vi "DAQ- Steper 2.vi"(0 "Travel (Degree)":dbl=100.0, 1 "Loda based":bool, 5 "Mode":i32(ring)=10178 items=["Finite Samples"=10178, "Continuous Samples"=10123, "Hardware Timed Single Point"=12522], 7 "Home Done":bool, 9 "Speed d/s":dbl=10.0, 11 "error in":errorcluster) -> (6 "Task Done Bit":bool, 15 "error out":errorcluster)   [LabVIEW 2020]
uses:
  Project Setup/Globle Variable/GR_Servo.vi
  <vilib>/DAQmx/create/channels.llb/DAQmx Create Channel (CO-Pulse Generation-Frequency).vi
  <vilib>/DAQmx/configure/timing.llb/DAQmx Timing (Implicit).vi
  Galobal variable_TI.vi
panel:
  out "32bit integer":i32
  in  "Motor PPR":dbl=3600.0
  in  "Motor Gear Ratio":dbl=1.0
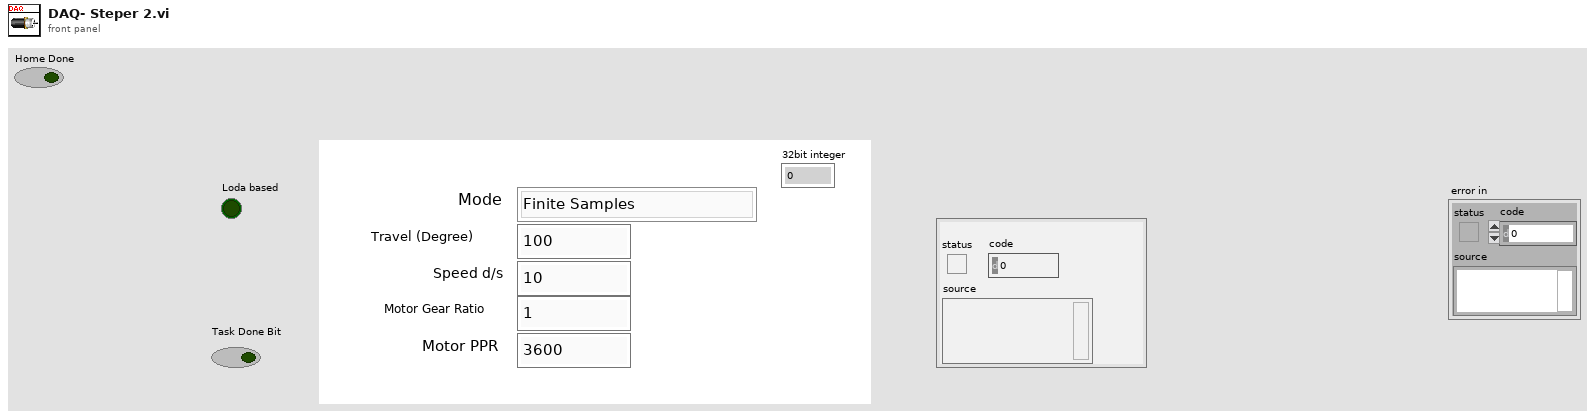
[diagram p1: front panel]
types:
  T1 = cluster{"MaxLoad ":dbl, "Min Load":dbl, "MaxDistance(mm)":dbl, "Min Distance(mm)":dbl, "Load Offset":dbl, "Model":string, "Difusser Code":string, "TFT Code ":string, "LVDT Offset":dbl}
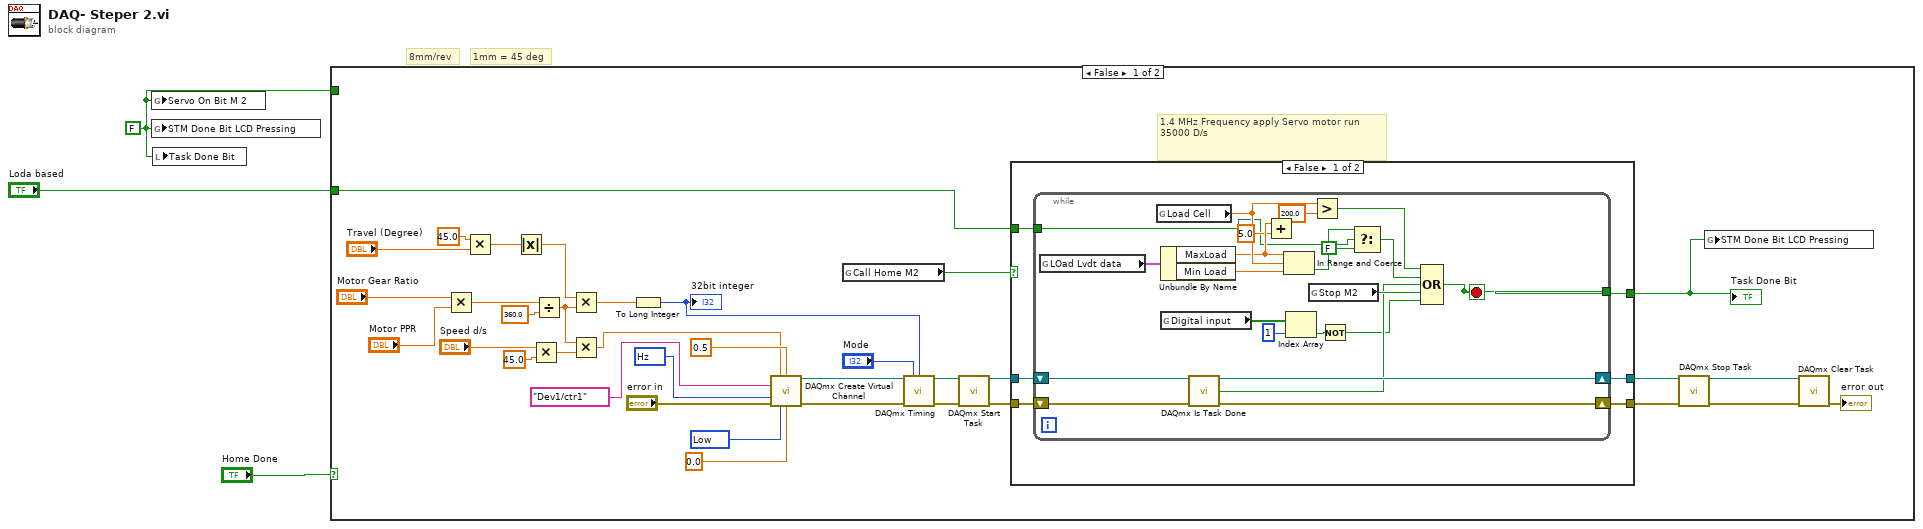
[diagram p0: block diagram]
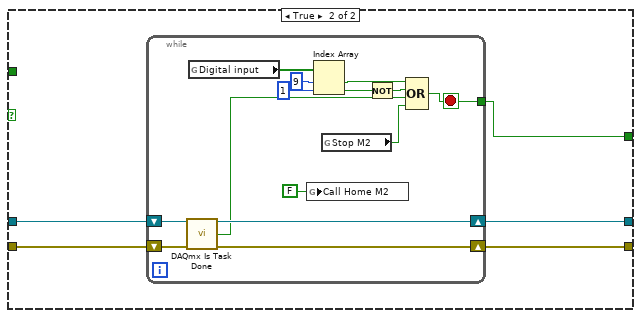
[diagram p2: hidden frame]
diagram:
  w3 = FALSE ("Servo On Bit M 2")
  # "1mm = 45 deg"
  # "8mm/rev"
  n1 = global write "GR_Servo.vi" "Servo On Bit M 2"(w3) -> ()
  n2 = global write "GR_Servo.vi" "STM Done Bit LCD Pressing"(w3) -> ()
  n3 = local write "Task Done Bit"(w3) -> ()
  n4 = case shown="False" "Home Done" {
    tunnel: w3 -> [_ _]
    tunnel: "Loda based" -> [w4 _]
    frame False {
      w18 = 10373 items=["Hz"=10373] ("units")
      w19 = 10214 items=["High"=10192, "Low"=10214] ("idle state")
      # "1.4 MHz Frequency apply Servo motor run \n35000 D/s"
      n5 = Multiply(x="Motor Gear Ratio", y="Motor PPR") -> (x*y=w28:dbl)
      n6 = Multiply(x=45.0, y="Travel (Degree)") -> (x*y=w16:dbl)
      n7 = Absolute Value(x=w16) -> (abs(x)=w27:dbl)
      n8 = Multiply(x="Speed d/s", y=45.0) -> (x*y=w13:dbl)
      n9 = Divide(x=w28, y=360.0) -> (x/y=w32:dbl)
      n10 = Multiply(x=w27, y=w32) -> (x*y=w17:dbl)
      n11 = Multiply(x=w32, y=w13) -> (x*y=w36:dbl)
      n12 = To Long Integer(number=w17) -> (32bit integer=w39:i32)
      "32bit integer" <- w39
      n13 = call-poly <vilib>:"DAQmx Create Virtual Channel.vi"("frequency"=w36, "duty cycle"=0.5, "counter"=tag "Dev1/ctr1", "units"=w18, "error in"="error in", "idle state"=w19, "initial delay"=0.0) -> ("task out"=w21:refnum<k21>, "error out"=w22:errorcluster)  [unwired: 7 in]
      n14 = global read "Galobal variable_TI.vi" "Call Home M2"() -> (w8:bool)
      n15 = call-poly <vilib>:"DAQmx Timing.vi"("task/channels in"=w21, "sample mode"="Mode", "samples per channel"=w39, "error in"=w22) -> ("task out"=w23:refnum<k21>, "error out"=w24:errorcluster)  [unwired: 10 in]
      n16 = call <vilib>:"DAQmx Start Task.vi"("task/channels in"=w23, "error in"=w24) -> ("task out"=w10:refnum<k21>, "error out"=w9:errorcluster)  [unwired: 12 in]
      n17 = case shown="False" w8 {
        tunnel: [w45 w69] -> w6
        tunnel: w10 -> [w44 w72]
        tunnel: [w43 w70] -> w7
        tunnel: w9 -> [w42 w71]
        tunnel: [w41 w68] -> w5
        tunnel: w4 -> [w40 _]
        frame False {
          n18 = while {
            shift-right: [w65] -> w43
            shift-left: w44 -> [w67]
            shift-right: [w66] -> w45
            shift-left: w42 -> [w64]
            tunnel: [w61] -> w41
            tunnel: w40 -> [w49]
            stop <- w61 stop-if-true
            n19 = global read "Galobal variable_TI.vi" "LOad Lvdt data"() -> (w56:T1)
            n20 = global read "Galobal variable_TI.vi" "Load Cell"() -> (w53:dbl)
            n21 = Unbundle By Name(w56) -> ("MaxLoad"=w52:dbl, "Min Load"=w55:dbl)
            n22 = global read "Galobal variable_TI.vi" "Digital input"() -> (w60:bool[])
            n23 = call <vilib>:"DAQmx Is Task Done.vi"("task/channels in"=w67, "error in"=w64) -> ("task out"=w65:refnum<k21>, "task done?"=w62:bool, "error out"=w66:errorcluster)  [unwired: 11 in]
            n24 = Add(x=w52, y=5.0) -> ()  [unwired: 1 out]
            n25 = In Range and Coerce(upper limit=w52, x=w53, lower limit=w55) -> (In Range?=w48:bool)  [unwired: 1 out]
            n26 = Index Array(array=w60, index=1) -> (element=w58:bool)
            n27 = global read "Galobal variable_TI.vi" "Stop M2"() -> (w63:bool)
            n28 = Greater?(x=w53, y=200.0) -> (0:w54:bool)
            n29 = Not(x=w58) -> (.not. x?=w57:bool)
            n30 = Select(t=w48, s=w49, f=FALSE) -> (s? t:f=w47:bool)
            n31 = Compound Arithmetic op=OR(w54, w47, w62, w63, w57) -> (w61:bool)
          }
        }
        frame True {
          n32 = while {
            shift-right: [w84] -> w70
            shift-left: w72 -> [w86]
            shift-right: [w85] -> w69
            shift-left: w71 -> [w83]
            tunnel: [w78] -> w68
            stop <- w78 stop-if-true
            n33 = call <vilib>:"DAQmx Is Task Done.vi"("task/channels in"=w86, "error in"=w83) -> ("task out"=w84:refnum<k21>, "task done?"=w79:bool, "error out"=w85:errorcluster)  [unwired: 11 in]
            n34 = global read "Galobal variable_TI.vi" "Digital input"() -> (w80:bool[])
            n35 = global write "Galobal variable_TI.vi" "Call Home M2"(FALSE ("Call Home M2")) -> ()
            n36 = Index Array(array=w80, index #1=9 ("index"), index #2=1 ("index")) -> (element #1=w75:bool, element #2=w74:bool)
            n37 = global read "Galobal variable_TI.vi" "Stop M2"() -> (w82:bool)
            n38 = Not(x=w74) -> (.not. x?=w73:bool)
            n39 = Compound Arithmetic op=OR(w75, w73, w79, w82) -> (w78:bool)
          }
        }
      }
      "Task Done Bit" <- w5
      n40 = call <vilib>:"DAQmx Stop Task.vi"("task/channels in"=w7, "error in"=w6) -> ("task out"=w25:refnum<k21>, "error out"=w35:errorcluster)  [unwired: 12 in]
      n41 = global write "GR_Servo.vi" "STM Done Bit LCD Pressing"(w5) -> ()
      n42 = call <vilib>:"DAQmx Clear Task.vi"("task in"=w25, "error in"=w35) -> ("error out"=→"error out":errorcluster)  [unwired: 13 in]
    }
    frame True {
    }
  }
